vi "Set 1553 Message Data.vi"(0 "MSG DATA In":u16[](array[numeric]), 5 "1553 Parameter":T1, 7 "Value":dbl, 11 "error in (no error)":errorcluster) -> (4 "MSG DATA Out":u16[](array[numeric]), 15 "error out":errorcluster)   [LabVIEW 2014]
uses:
  Controls/1553 Param.ctl
  AIT 1553 Custom Device.lvlib
panel:
  out "(hi.lo) 2":i16
  out "(hi.lo)":i32
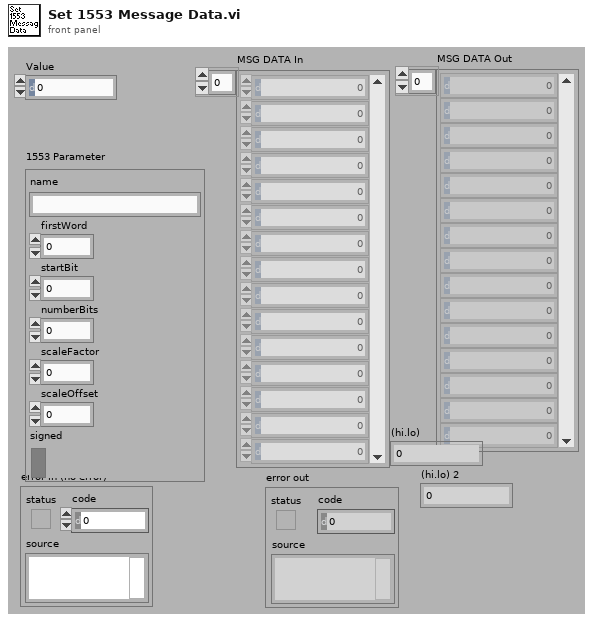
[diagram p1: front panel]
types:
  T1 = typedef "AIT 1553 Custom Device.lvlib/1553 Param.ctl" = cluster{"name":string, "firstWord":i32, "startBit":i32, "numberBits":i32, "scaleFactor":dbl, "scaleOffset":dbl, "signed":bool}
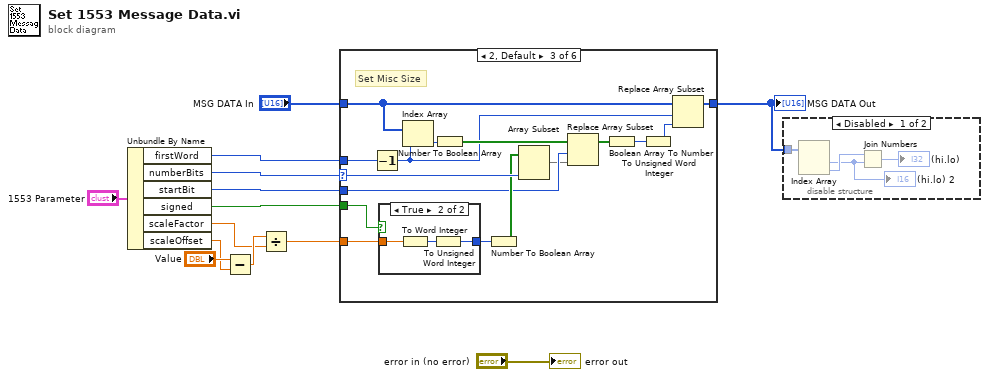
[diagram p0: block diagram]
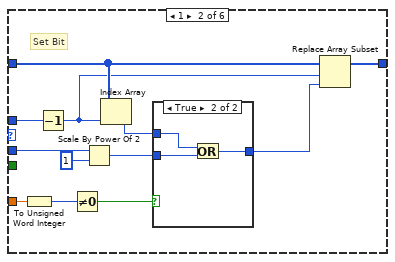
[diagram p3: hidden frame]
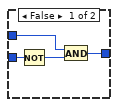
[diagram p4: hidden frame]
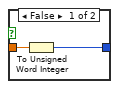
[diagram p5: hidden frame]
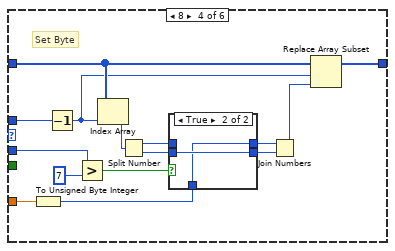
[diagram p6: hidden frame]
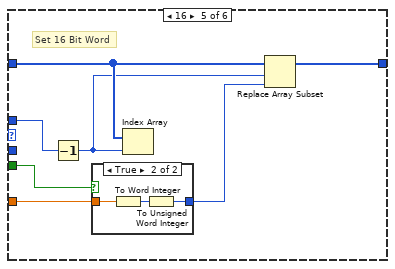
[diagram p8: hidden frame]
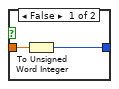
[diagram p9: hidden frame]
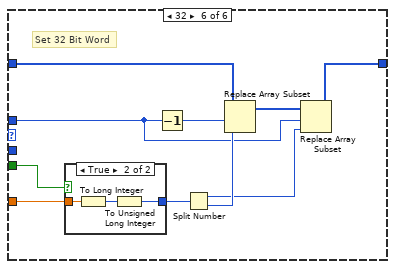
[diagram p10: hidden frame]
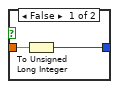
[diagram p11: hidden frame]
diagram:
  n1 = Unbundle By Name("1553 Parameter") -> ("firstWord"=w11:i32, "numberBits"=w10:i32, "startBit"=w9:i32, "signed"=w8:bool, "scaleFactor"=w4:dbl, "scaleOffset"=w5:dbl)
  n2 = Subtract(x="Value", y=w5) -> (x-y=w7:dbl)
  n3 = Divide(x=w7, y=w4) -> (x/y=w3:dbl)
  n4 = case shown="2, Default" w10 {
    selector: w10 -> [_ _ w45 _ _ _]
    tunnel: "MSG DATA In" -> [w14 w23 w37 w62 w79 w93]
    tunnel: w11 -> [_ w26 w46 w69 w80 w87]
    tunnel: w9 -> [_ w24 w41 w63 _ _]
    tunnel: w8 -> [_ _ w48 _ w76 w91]
    tunnel: w3 -> [_ w21 w49 w59 w77 w95]
    tunnel: [w14 w20 w35 w61 w74 w86] -> w1
    frame 0 {
      # "No Bits - Should not happen"
    }
    frame 1 {
      # "Set Bit"
      n5 = To Unsigned Word Integer(number=w21) -> (unsigned 16bit integer=w19:u16)
      n6 = Decrement(x=w26) -> (x-1=w22:i32)
      n7 = Not Equal To 0?(x=w19) -> (x != 0?=w18:bool)
      n8 = Scale By Power Of 2(n=w24, x=u16 1) -> (x*2^n=w16:u16)
      n9 = Index Array(array=w23, index=w22) -> (element=w17:u16)
      n10 = case shown="True" w18 {
        tunnel: w17 -> [w28 w31]
        tunnel: w16 -> [w30 w33]
        tunnel: [w27 w32] -> w15
        frame False {
          n11 = Not(x=w30) -> (.not. x?=w29:u16)
          n12 = And(x=w28, y=w29) -> (x .and. y?=w27:u16)
        }
        frame True {
          n13 = Or(x=w31, y=w33) -> (x .or. y?=w32:u16)
        }
      }
      n14 = Replace Array Subset(array=w23, new element=w15, index=w22) -> (w20:u16[])
    }
    frame 2, Default {
      # "Set Misc Size"
      n15 = Decrement(x=w46) -> (x-1=w36:i32)
      n16 = case shown="True" w48 {
        tunnel: w49 -> [w51 w54]
        tunnel: [w50 w52] -> w44
        frame False {
          n17 = To Unsigned Word Integer(number=w51) -> (unsigned 16bit integer=w50:u16)
        }
        frame True {
          n18 = To Word Integer(number=w54) -> (16bit integer=w53:i16)
          n19 = To Unsigned Word Integer(number=w53) -> (unsigned 16bit integer=w52:u16)
        }
      }
      n20 = Index Array(array=w37, index=w36) -> (element=w47:u16)
      n21 = Number To Boolean Array(number=w47) -> (Boolean array=w42:bool[])
      n22 = Number To Boolean Array(number=w44) -> (Boolean array=w43:bool[])
      n23 = Array Subset(array=w43, length=w45) -> (w40:bool[])  [unwired: 1 in]
      n24 = Replace Array Subset(array=w42, new element=w40, index=w41) -> (w38:bool[])
      n25 = Boolean Array To Number(Boolean array=w38) -> (number=w39:u32)
      n26 = To Unsigned Word Integer(number=w39) -> (unsigned 16bit integer=w34:u16)
      n27 = Replace Array Subset(array=w37, new element=w34, index=w36) -> (w35:u16[])
    }
    frame 8 {
      # "Set Byte"
      n28 = To Unsigned Byte Integer(number=w59) -> (unsigned 8bit integer=w58:u8)
      n29 = Decrement(x=w69) -> (x-1=w60:i32)
      n30 = Greater?(x=w63, y=u16 7) -> (0:w66:bool)
      n31 = Index Array(array=w62, index=w60) -> (element=w67:u16)
      n32 = Split Number(x=w67) -> (hi(x)=w65:u8, lo(x)=w64:u8)
      n33 = case shown="True" w66 {
        tunnel: w65 -> [w71 _]
        tunnel: w64 -> [_ w73]
        tunnel: [w71 w72] -> w57
        tunnel: w58 -> [w70 w72]
        tunnel: [w70 w73] -> w56
        frame False {
        }
        frame True {
        }
      }
      n34 = Join Numbers(hi=w57, lo=w56) -> ((hi.lo)=w55:u16)
      n35 = Replace Array Subset(array=w62, new element=w55, index=w60) -> (w61:u16[])
    }
    frame 16 {
      # "Set 16 Bit Word"
      n36 = Decrement(x=w80) -> (x-1=w78:i32)
      n37 = case shown="True" w76 {
        tunnel: w77 -> [w82 w85]
        tunnel: [w81 w83] -> w75
        frame False {
          n38 = To Unsigned Word Integer(number=w82) -> (unsigned 16bit integer=w81:u16)
        }
        frame True {
          n39 = To Word Integer(number=w85) -> (16bit integer=w84:i16)
          n40 = To Unsigned Word Integer(number=w84) -> (unsigned 16bit integer=w83:u16)
        }
      }
      n41 = Index Array(array=w79, index=w78) -> ()  [unwired: 1 out]
      n42 = Replace Array Subset(array=w79, new element=w75, index=w78) -> (w74:u16[])
    }
    frame 32 {
      # "Set 32 Bit Word"
      n43 = case shown="True" w91 {
        tunnel: w95 -> [w97 w100]
        tunnel: [w96 w98] -> w94
        frame False {
          n44 = To Unsigned Long Integer(number=w97) -> (unsigned 32bit integer=w96:u32)
        }
        frame True {
          n45 = To Long Integer(number=w100) -> (32bit integer=w99:i32)
          n46 = To Unsigned Long Integer(number=w99) -> (unsigned 32bit integer=w98:u32)
        }
      }
      n47 = Decrement(x=w87) -> (x-1=w92:i32)
      n48 = Split Number(x=w94) -> (hi(x)=w88:u16, lo(x)=w90:u16)
      n49 = Replace Array Subset(array=w93, new element=w90, index=w92) -> (w89:u16[])
      n50 = Replace Array Subset(array=w89, new element=w88, index=w87) -> (w86:u16[])
    }
  }
  "MSG DATA Out" <- w1
  n51 = disable-structure shown="Disabled" {
    disable-tunnel: w1 -> [w104 _]
    frame Disabled {
      n52 = Index Array(array=w104) -> (element #1=w101:u16, element #2=w103:u16)  [unwired: 2 in]
      "(hi.lo) 2" <- w101
      n53 = Join Numbers(hi=w103, lo=w101) -> ((hi.lo)=→"(hi.lo)":u32)
    }
    frame Enabled {
    }
  }
  "error out" <- "error in (no error)"
